vi "AerotechPosition.vi"(0 "error in (no error)":errorcluster, 5 "Position":dbl) -> (3 "error out":errorcluster)   [LabVIEW 2009]
uses:
  Controls/AerotechCommand.ctl
  Controls/AerotechTarget.ctl
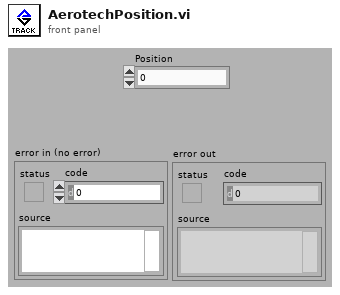
[diagram p1: front panel]
types:
  T1 = typedef "AerotechTarget.ctl" = cluster{"Time":timestamp, "Position":dbl, "Velocity":dbl}
  T2 = typedef "AerotechCommand.ctl" = enum16{"TRACK", "POSITION", "STOP", "HOME", "QUIT"}
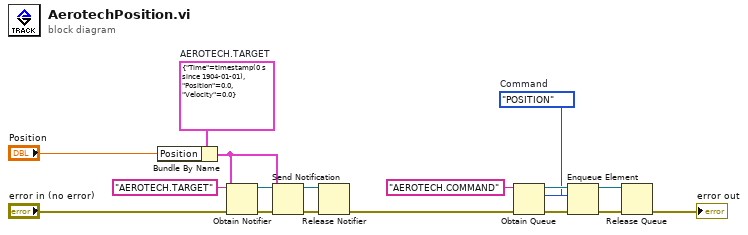
[diagram p0: block diagram]
diagram:
  w8 = T1 {"Time"=timestamp(0 s since 1904-01-01), "Position"=0.0, "Velocity"=0.0}  # AEROTECH.TARGET
  w14 = AerotechCommand."POSITION"  # Command
  n1 = Bundle By Name(cluster=w8, "Position"="Position") -> (w4:T1)
  n2 = Obtain Notifier(name (unnamed)="AEROTECH.TARGET", notification data type=w4, error in (no error)="error in (no error)") -> (notifier out=w6:refnum<notifier>, error out=w5:errorcluster)  [unwired: 1 in, 1 out]
  n3 = Send Notification(notification=w4, notifier=w6, error in (no error)=w5) -> (notifier out=w3:refnum<notifier>, error out=w2:errorcluster)
  n4 = Release Notifier(notifier=w3, error in (no error)=w2) -> (error out=w1:errorcluster)  [unwired: 1 in, 2 out]
  n5 = Obtain Queue(name (unnamed)="AEROTECH.COMMAND", element data type=w14, error in (no error)=w1) -> (queue out=w15:refnum<queue>, error out=w16:errorcluster)  [unwired: 2 in, 1 out]
  n6 = Enqueue Element(queue=w15, element=w14, error in (no error)=w16) -> (queue out=w12:refnum<queue>, error out=w13:errorcluster)  [unwired: 1 in, 1 out]
  n7 = Release Queue(queue=w12, error in (no error)=w13) -> (error out=→"error out":errorcluster)  [unwired: 1 in, 2 out]
